vi "CanMove.vi"(0 "Chessboard in":T2, 5 "ItemIndex":T1, 7 "StoneColor":u16, 11 "error in (no error)":errorcluster) -> (4 "Chessboard out":T2, 6 "ItemIndex out":T1, 8 "StoneColor out":u16, 10 "CanMove?":bool, 15 "error out":errorcluster)   [LabVIEW 2009]
doc: "To check if the position can move stone."
uses:
  Controls/Chess.ctl
  Controls/ItemIndex.ctl
  Controls/directions.ctl
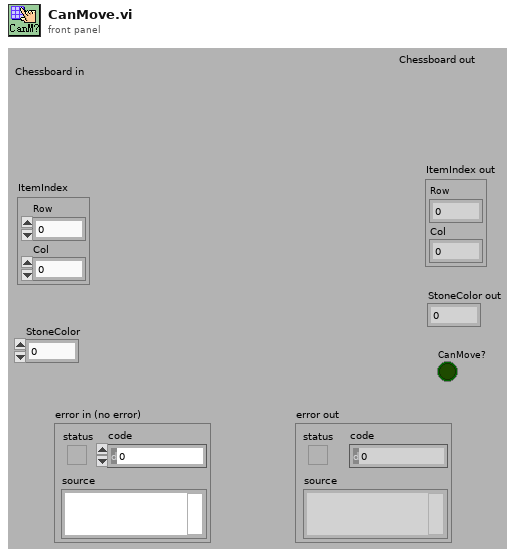
[diagram p1: front panel]
types:
  T1 = typedef "ItemIndex.ctl" = cluster{"Row":i32, "Col":i32}
  T2 = typedef "Chess.ctl" = u16[][]
  T3 = typedef "directions.ctl" = enum16{"Left", "Right", "Top", "Bottom", "TopLeft", "TopRight", "BottomLeft", "BottomRight", "ClearAll", "ReadAll"}
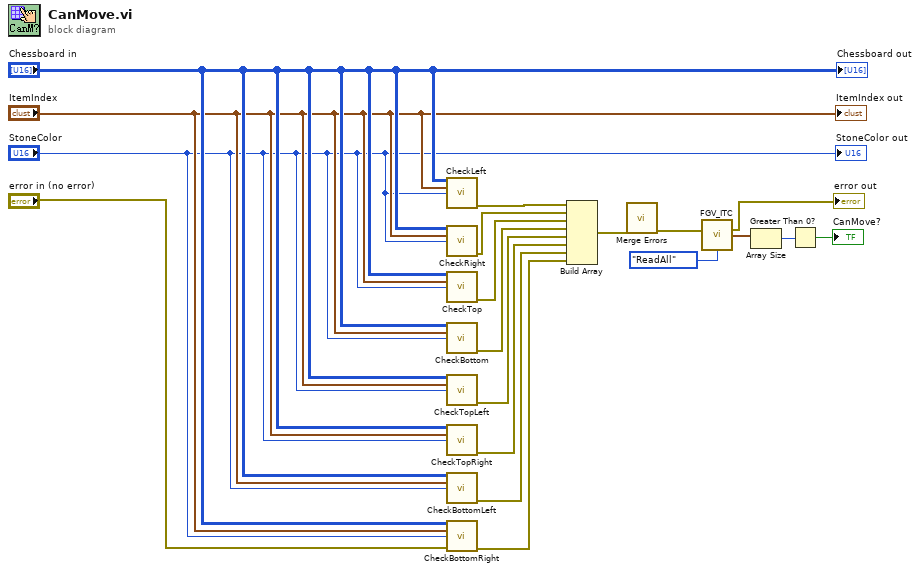
[diagram p0: block diagram]
diagram:
  n1 = call "CheckLeft.vi"("Chessboard"="Chessboard in", "ItemIndex"="ItemIndex", "StoneColor"="StoneColor") -> ("error out"=w16:errorcluster)  [unwired: 12 in]
  n2 = call "CheckRight.vi"("Chessboard"="Chessboard in", "ItemIndex"="ItemIndex", "StoneColor"="StoneColor") -> ("error out"=w15:errorcluster)  [unwired: 12 in]
  n3 = call "CheckTop.vi"("Chessboard"="Chessboard in", "ItemIndex"="ItemIndex", "StoneColor"="StoneColor") -> ("error out"=w14:errorcluster)  [unwired: 12 in]
  n4 = call "CheckBottom.vi"("Chessboard"="Chessboard in", "ItemIndex"="ItemIndex", "StoneColor"="StoneColor") -> ("error out"=w13:errorcluster)  [unwired: 12 in]
  n5 = call "CheckTopLeft.vi"("Chessboard"="Chessboard in", "ItemIndex"="ItemIndex", "StoneColor"="StoneColor") -> ("error out"=w12:errorcluster)  [unwired: 12 in]
  n6 = call "CheckTopRight.vi"("Chessboard"="Chessboard in", "ItemIndex"="ItemIndex", "StoneColor"="StoneColor") -> ("error out"=w11:errorcluster)  [unwired: 12 in]
  n7 = call "CheckBottomLeft.vi"("Chessboard"="Chessboard in", "ItemIndex"="ItemIndex", "StoneColor"="StoneColor") -> ("error out"=w10:errorcluster)  [unwired: 12 in]
  n8 = call "CheckBottomRight.vi"("Chessboard"="Chessboard in", "ItemIndex"="ItemIndex", "StoneColor"="StoneColor", "error in (no error)"="error in (no error)") -> ("error out"=w9:errorcluster)  [unwired: 11 in]
  n9 = Build Array(w16, w15, w14, w13, w12, w11, w10, w9) -> (w7:errorcluster[])
  n10 = call <vilib>:"Merge Errors.vi"("error array in"=w7) -> ("error out"=w6:errorcluster)  [unwired: 6 in]
  n11 = call "FGV_ITC.vi"("error in (no error)"=w6, "Action"=directions."ReadAll") -> ("error out"=→"error out":errorcluster, "ItemsToChange"=w4:T1[])  [unwired: 12 in]
  n12 = Array Size(array=w4) -> (size(s)=w3:i32)
  n13 = Greater Than 0?(x=w3) -> (x > 0?=→"CanMove?":bool)
  "Chessboard out" <- "Chessboard in"
  "ItemIndex out" <- "ItemIndex"
  "StoneColor out" <- "StoneColor"
